vi "GC Vacuum - Step 6.vi"(7 "Step":i32, 8 "error in":errorcluster, 9 "Test Results In":T8, 10 "Gas":T1, 11 "GC Configuration":T2) -> (0 "error out":errorcluster, 1 "Test Results Out":T8, 2 "Gas Out":T1 caption="Gas", 3 "GC Configuration Out":T2)   [LabVIEW 2015]
uses:
  Controls/Test Information.ctl
  Controls/Vacuum Test.ctl
  Controls/Test Timing.ctl
  Controls/Vaccum Thresholds.ctl
  Controls/Helium Test.ctl
  Controls/Helium Thresholds.ctl
  CAN Communication/Gas/Typedefs/Session Handle.ctl
  CAN Communication/Gas/Gas.lvclass
  Controls/Test Results.ctl
  Controls/Step Result.ctl
  CAN Communication/Gas/Typedefs/Valves.ctl
  SubVIs/Timing/Timing.lvlib
  User Interface/UI Handler/UI Handler.lvclass
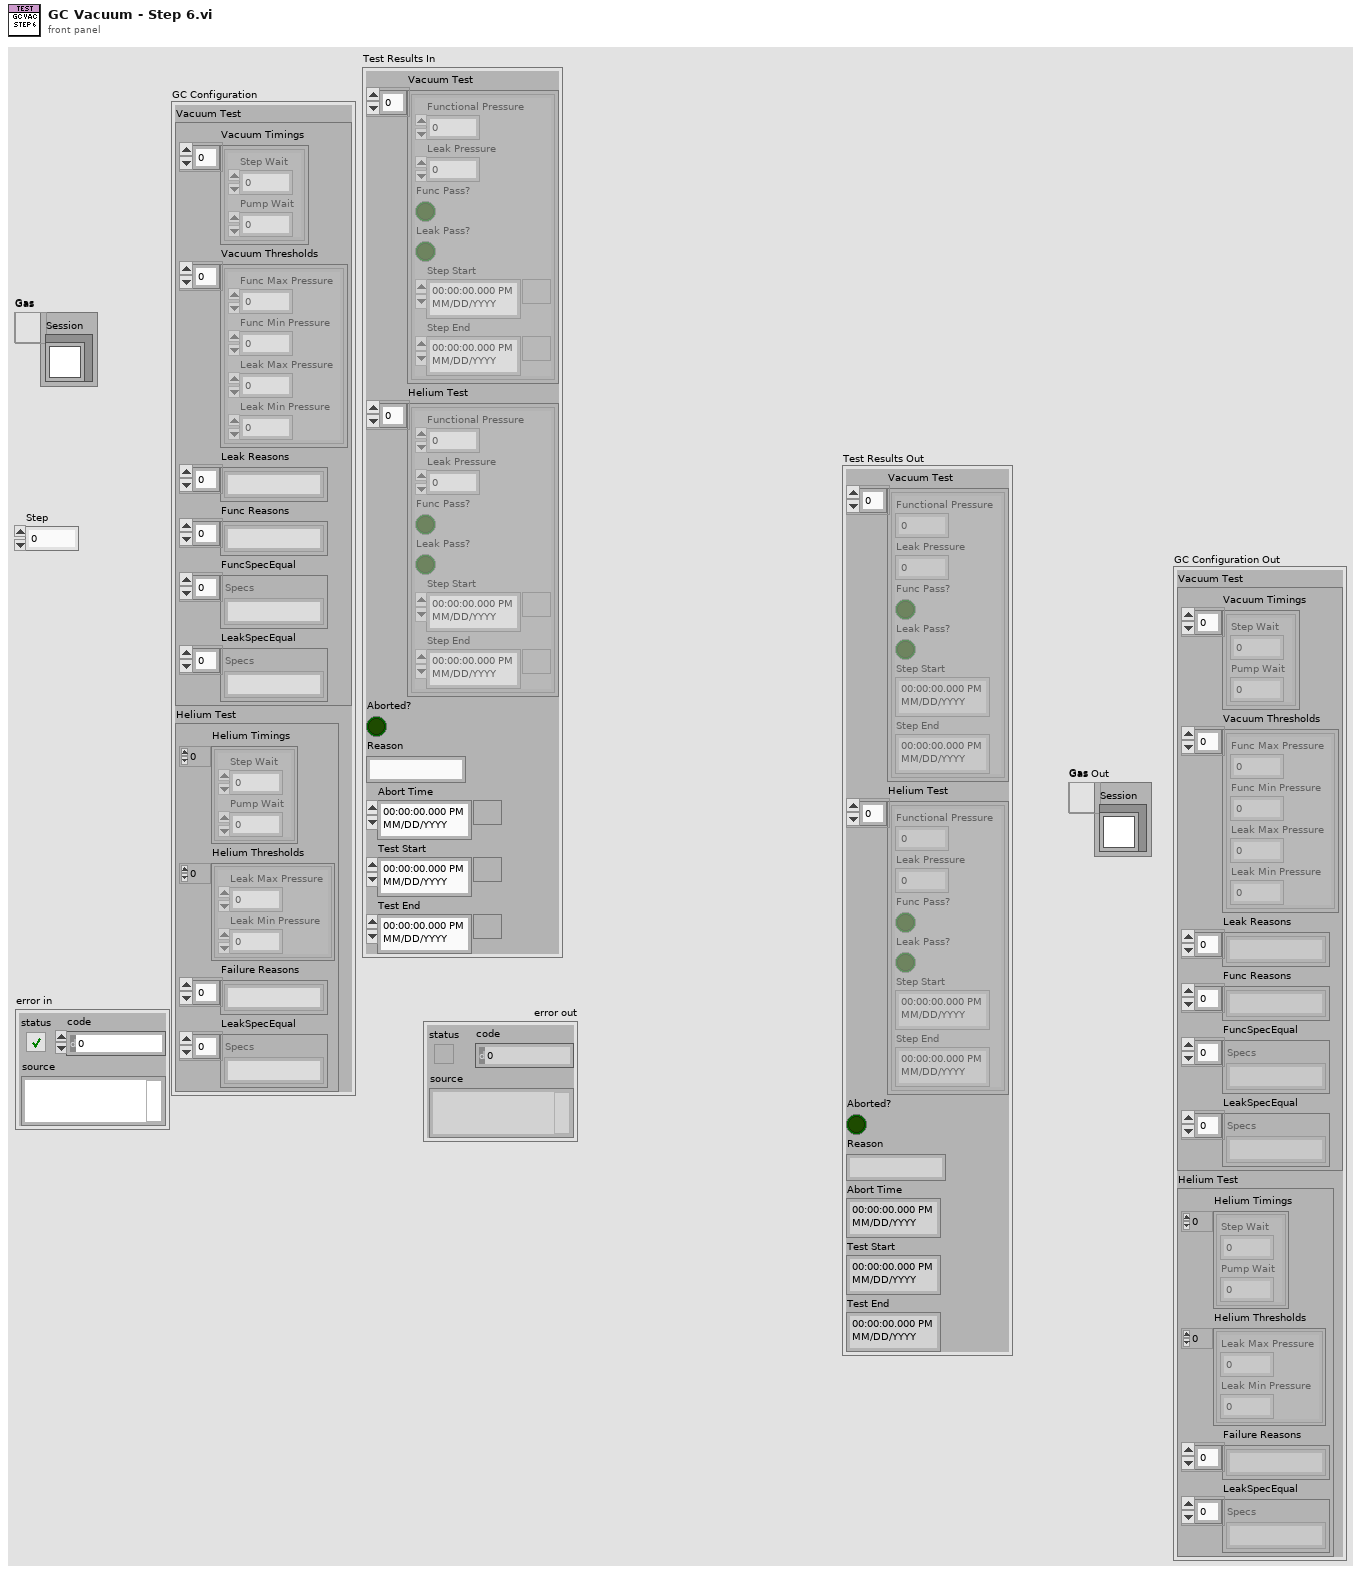
[diagram p1: front panel]
types:
  T1 = typedef "Gas.lvclass/Session Handle.ctl" = refnum<data-value>
  T2 = typedef "Test Information.ctl" = cluster{"Vacuum Test":T3, "Helium Test":T6}
  T3 = typedef "Vacuum Test.ctl" = cluster{"Vacuum Timings":T4[], "Vacuum Thresholds":T5[], "Leak Reasons":string[], "Func Reasons":string[], "FuncSpecEqual":string[], "LeakSpecEqual":string[]}
  T4 = typedef "Test Timing.ctl" = cluster{"Step Wait":dbl, "Pump Wait":dbl}
  T5 = typedef "Vaccum Thresholds.ctl" = cluster{"Func Max Pressure":dbl, "Func Min Pressure":dbl, "Leak Max Pressure":dbl, "Leak Min Pressure":dbl}
  T6 = typedef "Helium Test.ctl" = cluster{"Helium Timings":T4[], "Helium Thresholds":T7[], "Failure Reasons":string[], "LeakSpecEqual":string[]}
  T7 = typedef "Helium Thresholds.ctl" = cluster{"Leak Max Pressure":dbl, "Leak Min Pressure":dbl}
  T8 = typedef "Test Results.ctl" = cluster{"Vacuum Test":T9[], "Helium Test":T9[], "Aborted?":bool, "Reason":string, "Abort Time":timestamp, "Test Start":timestamp, "Test End":timestamp}
  T9 = typedef "Step Result.ctl" = cluster{"Functional Pressure":dbl, "Leak Pressure":dbl, "Func Pass?":bool, "Leak Pass?":bool, "Step Start":timestamp, "Step End":timestamp}
  T10 = typedef "Gas.lvclass/Valves.ctl" = u16
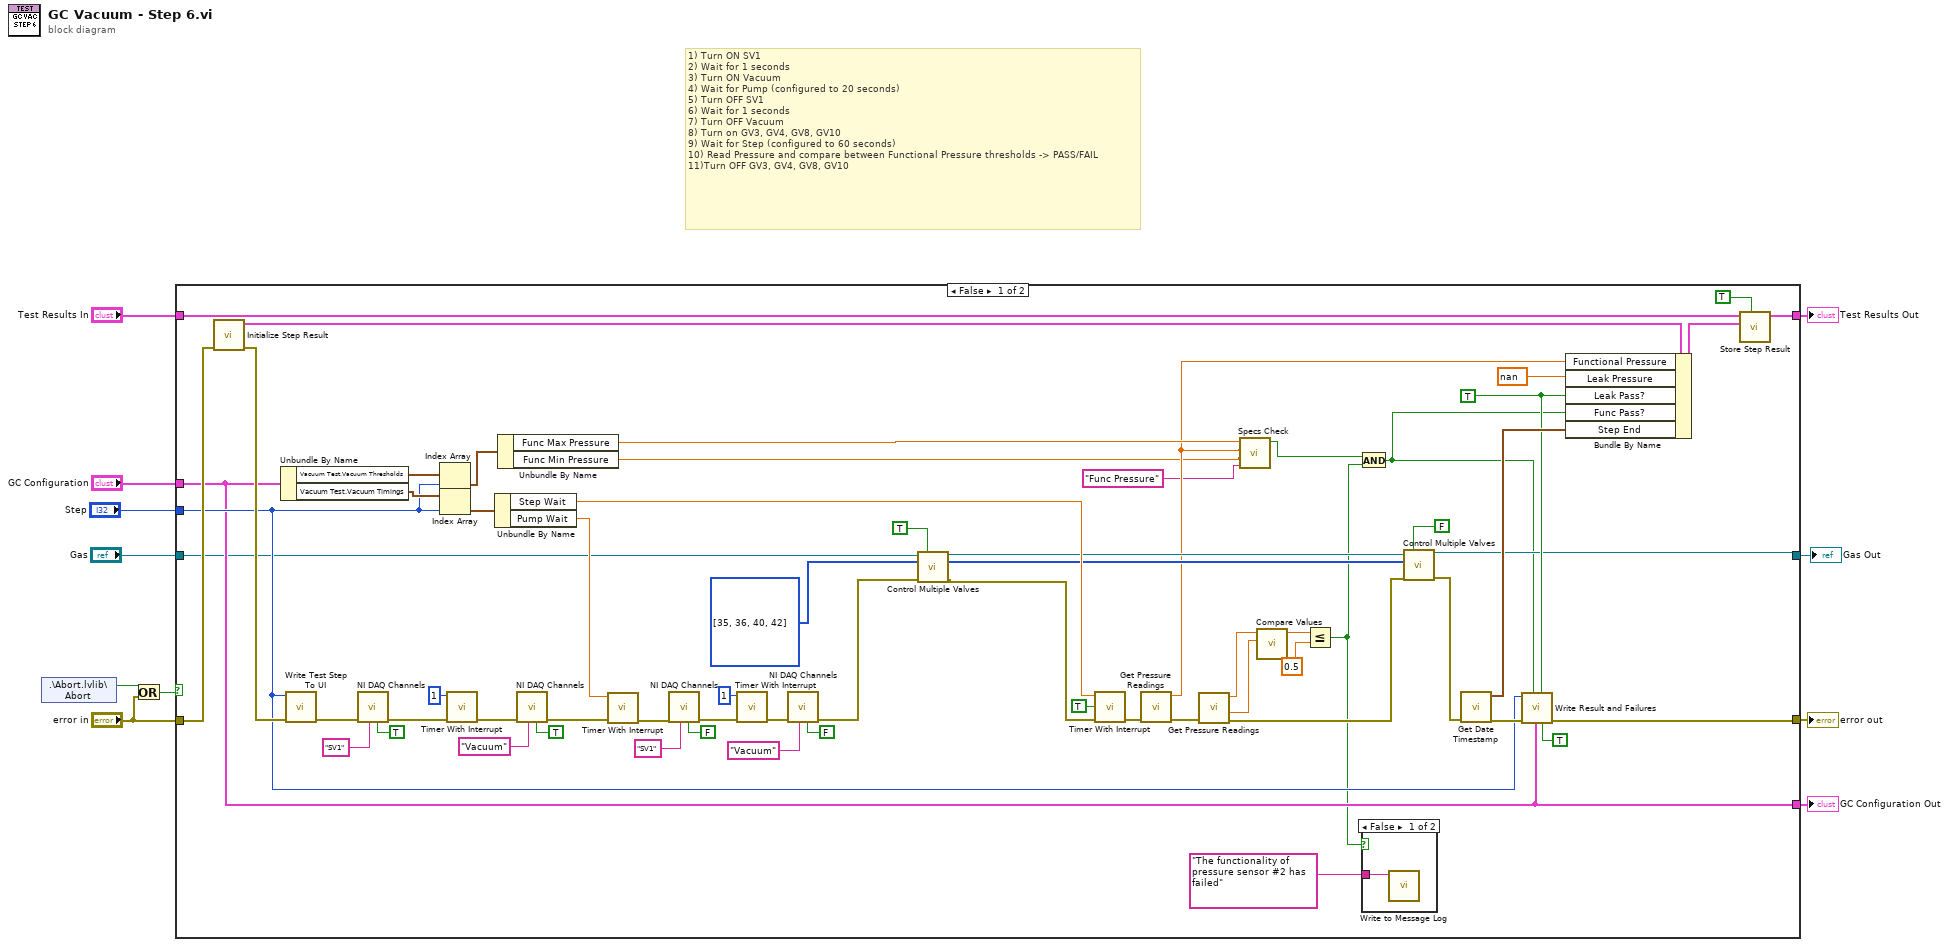
[diagram p0: block diagram]
diagram:
  # "1) Turn ON SV1\n2) Wait for 1 seconds\n3) Turn ON Vacuum\n4) Wait for Pump (configured to 20 seconds)\n5) Turn OFF SV1\n6) Wait for 1 seconds\n7) Turn OFF Vacuum\n8) Turn on GV3, GV4, GV8, GV10\n9) Wait for Step (configured to 60 seconds)\n10) Read Pressure and compare between Functional Pressure thresholds -> PASS/FAIL\n11)Turn OFF GV3, GV4, GV8, GV10"
  n1 = shared-variable ".\\Abort.lvlib\\Abort"() -> (w10:bool)  [unwired: 1 in, 1 out]
  n2 = Or(x=w10, y="error in") -> (x .or. y?=w9:bool)
  n3 = case shown="False" w9 {
    tunnel: "error in" -> [w75 w79]
    tunnel: "Test Results In" -> [w72 w80]
    tunnel: [w73 w80] -> w7
    tunnel: [w60 w79] -> w6
    tunnel: "GC Configuration" -> [w58 w78]
    tunnel: "Step" -> [w59 _]
    tunnel: [w58 w78] -> w3
    tunnel: [w47 w77] -> w1
    tunnel: "Gas" -> [w52 w77]
    frame False {
      w51 = T10[] [35, 36, 40, 42] items=["GV1"=33, "GV2"=34, "GV3"=35, "GV4"=36, "GV5"=37, "GV6"=38, "GV7"=39, "GV8"=40, "GV9"=41, "GV10"=42, "GV11"=43, "LV3"=51, "LV4"=52]
      w54 = TRUE ("Leak Pass?")
      n4 = call "Initialize Step Result.vi"("error in (no error)"=w75) -> ("error out"=w74:errorcluster, "New Step Result"=w71:T9)  [unwired: 8 in, 1 out]
      n5 = Unbundle By Name(w58) -> ("Vacuum Test.Vacuum Thresholds"=w68:T5[], "Vacuum Test.Vacuum Timings"=w67:T4[])
      n6 = call "Write Test Step To UI.vi"("error in (no error)"=w74, "Step"=w59) -> ("error out"=w41:errorcluster)  [unwired: 9 in]
      n7 = call "NI DAQ Channels.vi"("Control"=TRUE ("State"), "Channel"="SV1", "error in (no error)"=w41) -> ("error out"=w40:errorcluster)  [unwired: 7 in, 1 out]
      n8 = Index Array(array=w68, index=w59) -> (element=w65:T5)
      n9 = Index Array(array=w67, index=w59) -> (element=w66:T4)
      n10 = call "Timer With Interrupt.vi"("error in (no error)"=w40, "Wait (s)"=1) -> ("error out"=w38:errorcluster)  [unwired: 7 in, 2 out]
      n11 = Unbundle By Name(w66) -> ("Step Wait"=w64:dbl, "Pump Wait"=w56:dbl)
      n12 = Unbundle By Name(w65) -> ("Func Max Pressure"=w15:dbl, "Func Min Pressure"=w13:dbl)
      n13 = call "NI DAQ Channels.vi"("Control"=TRUE ("State"), "Channel"="Vacuum", "error in (no error)"=w38) -> ("error out"=w37:errorcluster)  [unwired: 7 in, 1 out]
      n14 = call "Timer With Interrupt.vi"("error in (no error)"=w37, "Wait (s)"=w56) -> ("error out"=w35:errorcluster)  [unwired: 7 in, 2 out]
      n15 = call "NI DAQ Channels.vi"("Control"=FALSE ("State"), "Channel"="SV1", "error in (no error)"=w35) -> ("error out"=w34:errorcluster)  [unwired: 7 in, 1 out]
      n16 = call "Timer With Interrupt.vi"("error in (no error)"=w34, "Wait (s)"=1) -> ("error out"=w32:errorcluster)  [unwired: 7 in, 2 out]
      n17 = call "NI DAQ Channels.vi"("Control"=FALSE ("State"), "Channel"="Vacuum", "error in (no error)"=w32) -> ("error out"=w31:errorcluster)  [unwired: 7 in, 1 out]
      n18 = call "Control Multiple Valves.vi"("Session Handle in"=w52, "Energize?"=TRUE, "Valves"=w51, "error in (no error)"=w31) -> ("Session Handle out"=w48:T1, "Valves Out"=w46:T10[], "error out"=w49:errorcluster)  [unwired: 8 in, 1 out]
      n19 = call "Timer With Interrupt.vi"("error in (no error)"=w49, "Update UI?"=TRUE, "Wait (s)"=w64) -> ("error out"=w62:errorcluster)  [unwired: 6 in, 2 out]
      n20 = call "Get Pressure Readings.vi"("error in (no error)"=w62) -> ("error out"=w30:errorcluster, "NI-DAQ Pressure"=w14:dbl)  [unwired: 6 in, 3 out]
      n21 = call "Get Pressure Readings.vi"("error in (no error)"=w30) -> ("error out"=w24:errorcluster, "GAS Pressure 2"=w28:dbl, "NI-DAQ Pressure"=w29:dbl)  [unwired: 6 in, 2 out]
      n22 = call "Specs Check.vi"("parameter"="Func Pressure", "lower limit"=w13, "x"=w14, "upper limit"=w15) -> ("In Range?"=w16:bool)  [unwired: 6 in, 1 out]
      n23 = call "Compare Values.vi"("P2"=w28, "P1"=w29) -> ("Abs Diff"=w27:dbl)  [unwired: 9 in]
      n24 = Less Or Equal?(x=w27, y=0.5) -> (x <= y?=w23:bool)
      n25 = And(x=w16, y=w23) -> (x .and. y?=w25:bool)
      n26 = case shown="False" w23 {
        tunnel: "The functionality of pressure sensor #2 has failed" ("Message") -> [w76 _]
        frame False {
          n27 = call "Write to Message Log.vi"("Message"=w76) -> ()  [unwired: 10 in, 1 out]
        }
        frame True {
        }
      }
      n28 = call "Control Multiple Valves.vi"("Session Handle in"=w48, "Energize?"=FALSE, "Valves"=w46, "error in (no error)"=w24) -> ("Session Handle out"=w47:T1, "error out"=w44:errorcluster)  [unwired: 8 in, 2 out]
      n29 = call "Get Date Timestamp.vi"("error in (no error)"=w44) -> ("error out"=w61:errorcluster, "current time"=w69:timestamp)  [unwired: 9 in]
      n30 = call "Write Result and Failures.vi"("Vacuum?"=TRUE, "Leak"=w54, "GC Configuration"=w58, "Func"=w25, "error in (no error)"=w61, "Step"=w59) -> ("error out"=w60:errorcluster)  [unwired: 5 in]
      n31 = Bundle By Name(cluster=w71, "Functional Pressure"=w14, "Leak Pressure"=nan ("Step Pressure"), "Leak Pass?"=w54, "Func Pass?"=w25, "Step End"=w69) -> (w70:T9)
      n32 = call "Store Step Result.vi"("Vacuum?"=TRUE, "Step Result"=w70, "Test Results In"=w72) -> ("Test Results Out"=w73:T8)  [unwired: 8 in]
    }
    frame True {
    }
  }
  "error out" <- w6
  "Test Results Out" <- w7
  "GC Configuration Out" <- w3
  "Gas Out" <- w1
